vi "Stop Core.vi"(10 "final error code":i32, 11 "BoundViewManager in":refnum<class "BoundViewManager.lvclass">) -> (3 "BoundViewManager out":refnum<class "BoundViewManager.lvclass">)   [LabVIEW 2017, in "BoundViewManager.lvlib" / "BoundViewManager.lvclass"]
doc: "(<B>Filename</B>: Actor Framework.lvlib:Actor.lvclass:Stop Core.vi)\n\nDefines what the actor does before it stops. Use the <B>final error code</B> input to determine whether the actor shut down in response to an error.\n\nBy default, this method does nothing. A descendant class may override it to define behavior, such as shutting down any processes the actor initiated in its override of the Actor Core method.\n\n<License>\nCopyright © 2017 Composed Systems, LLC | All rights reserved\nwww.composed.io\n\nAuthor: Ethan Stern <ethan.stern@composed.io>\n\nThis software is provided \"AS IS\" WITHOUT WARRANTIES, either express or implied, AND IS FOR EDUCATIONAL PURPOSES ONLY.\n</License>"
uses:
  <vilib>/gpm_packages/@cs/ViewManager/source/BoundViewManager/BoundViewManager.lvclass
  <vilib>/gpm_packages/@cs/ViewManager/source/BoundViewManager/BoundViewManager.lvclass/BoundViewManager.ctl
  <vilib>/gpm_packages/@cs/mva-viewable/Source/IViewManager/IViewManager/IViewManager.lvclass
  <vilib>/gpm_packages/@cs/mva-viewable/Source/IViewable/ProtectedSubpanel/ProtectedSubpanel.lvclass
  <vilib>/gpm_packages/@cs/lookup-table/Source/LookupTable/LookupTable.lvclass
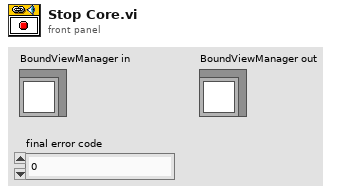
[diagram p1: front panel]
types:
  T1 = typedef "IViewable.lvlib/ProtectedSubpanel.lvclass/Protected Subpanel Reference.ctl" = refnum<data-value>
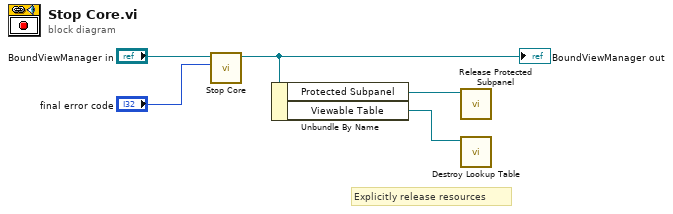
[diagram p0: block diagram]
diagram:
  # "Explicitly release resources"
  n1 = call-parent "Stop Core.vi"("final error code"="final error code", "IViewManager in"="BoundViewManager in") -> ("IViewManager out"=w3:refnum<class "BoundViewManager.lvclass">)  [unwired: 9 in]
  "BoundViewManager out" <- w3
  n2 = Unbundle By Name(w3) -> ("Protected Subpanel"=w2:T1, "Viewable Table"=w1:refnum<data-value>)
  n3 = call <vilib>:"Release Protected Subpanel.vi"("Protected Subpanel"=w2) -> ()  [unwired: 10 in, 1 out]
  n4 = call <vilib>:"Destroy Lookup Table.vi"("LookupTable Reference"=w1) -> ()  [unwired: 10 in, 1 out]
